vi "Auto Front Lift.vi"(9 "Encoder Input":dbl, 10 "Lower Range":dbl, 11 "Upper Range":dbl) -> (2 "Output":dbl)   [LabVIEW 2014]
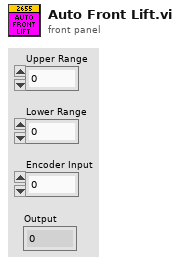
[diagram p1: front panel]
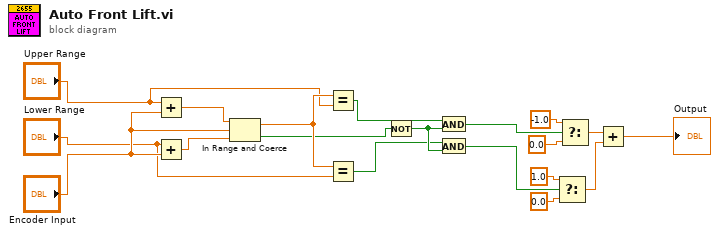
[diagram p0: block diagram]
diagram:
  n1 = Add(x="Upper Range", y="Encoder Input") -> (x+y=w18:dbl)
  n2 = Add(x="Lower Range", y="Encoder Input") -> (x+y=w19:dbl)
  n3 = In Range and Coerce(upper limit=w18, x="Encoder Input", lower limit=w19) -> (coerced(x)=w5:dbl, In Range?=w2:bool)
  n4 = Equal?(x=w5, y="Upper Range") -> (x = y?=w8:bool)
  n5 = Equal?(x=w5, y="Lower Range") -> (x = y?=w6:bool)
  n6 = Not(x=w2) -> (.not. x?=w7:bool)
  n7 = And(x=w8, y=w7) -> (x .and. y?=w10:bool)
  n8 = And(x=w6, y=w7) -> (x .and. y?=w9:bool)
  n9 = Select(t=1.0, s=w9, f=0.0) -> (s? t:f=w11:dbl)
  n10 = Select(t=-1.0, s=w10, f=0.0) -> (s? t:f=w12:dbl)
  n11 = Add(x=w12, y=w11) -> (x+y=→"Output":dbl)
